vi "add scan time(SubVI).vi"(10 "字符串":string) -> (1 "ok or cancel":bool, 2 "连接的字符串":string)   [LabVIEW 2019, in "Add Seq.lvlib"]
uses:
  Add Seq.lvlib
panel:
  in  "steps":i32
  in  "total time":dbl
  in  "cancel":bool
  in  "ok":bool
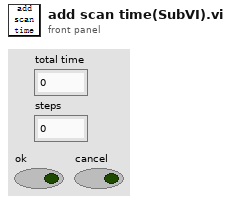
[diagram p1: front panel]
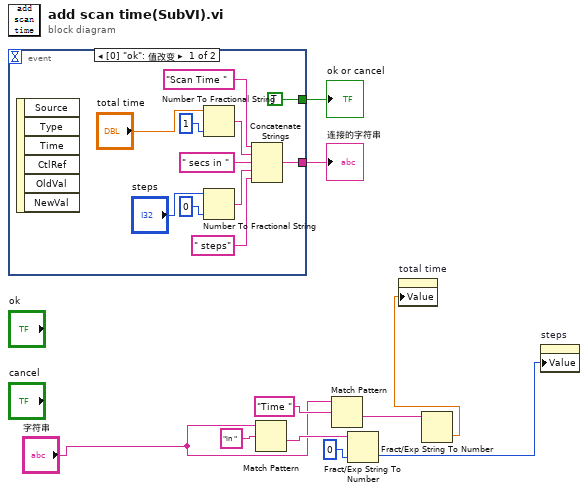
[diagram p0: block diagram]
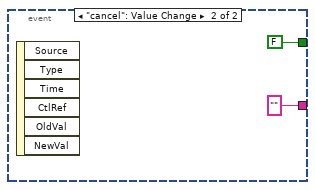
[diagram p2: hidden frame]
diagram:
  n1 = event shown="[0] \"ok\": 值改变" {
    selector: _ -> [_ _]
    dyn-events: _ -> [_ _]
    timeout: _ -> [_ _]
    tunnel: [TRUE FALSE] -> w10
    tunnel: [w11 "" ("分隔符")] -> w9
    event "ok": Value Change {
      n2 = event-data() -> ()  [unwired: 1 in, 6 out]
      n3 = Number To Fractional String(number="total time", precision (6)=i16 1 ("精度(6)")) -> (F-format string=w18:string)  [unwired: 2 in]
      n4 = Number To Fractional String(number="steps", precision (6)=i16 0 ("精度(6)")) -> (F-format string=w13:string)  [unwired: 2 in]
      n5 = Concatenate Strings("Scan Time " ("字符串"), w18, " secs in " ("字符串"), w13, " steps" ("字符串")) -> (w11:string)
    }
    event "cancel": Value Change {
      n6 = event-data() -> ()  [unwired: 1 in, 6 out]
    }
  }
  "ok or cancel" <- w10
  "连接的字符串" <- w9
  n7 = Match Pattern(string="字符串", regular expression="in " ("正则表达式")) -> (after substring=w5:string)  [unwired: 1 in, 3 out]
  n8 = Match Pattern(string="字符串", regular expression="Time " ("正则表达式")) -> (after substring=w7:string)  [unwired: 1 in, 3 out]
  n9 = Fract/Exp String To Number(string=w5, default (0 dbl)=0) -> (number=w2:i32)  [unwired: 2 in, 1 out]
  n10 = Fract/Exp String To Number(string=w7) -> (number=w1:dbl)  [unwired: 3 in, 1 out]
  n11 = property on="total time" class="DigNum (严格)"("Value"=w1) -> ()  [unwired: 2 in, 2 out]
  n12 = property on="steps" class="DigNum (严格)"("Value"=w2) -> ()  [unwired: 2 in, 2 out]
